vi "Untitled 1.vi"() -> ()   [LabVIEW 2015]
uses:
  <vilib>/measure/NI_MAPro.lvlib
  <vilib>/measure/mamon.llb/Waveform Peak Detection for 1 Chan.vi
  <vilib>/Analysis/NI_AALBase.lvlib
  <vilib>/Analysis/baseanly.llb/Mean (DBL).vi
panel:
  in  "subarray":i32[](array[numeric])
  out "Locations":dbl[](array[numeric]) format="%.2p"
  out "Waveform Chart":i32[](graph)
  out "size(s)":i32
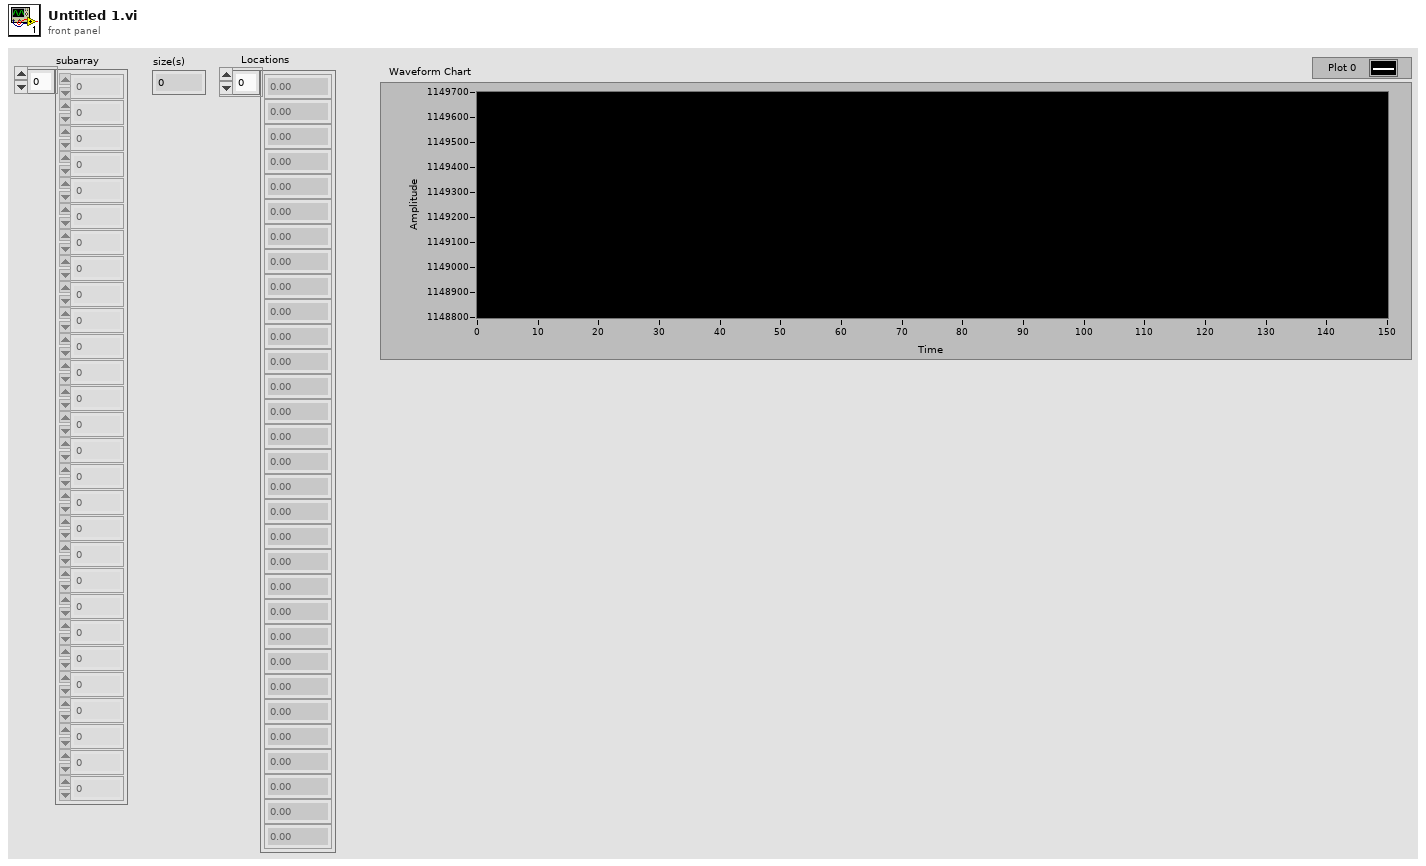
[diagram p1: front panel]
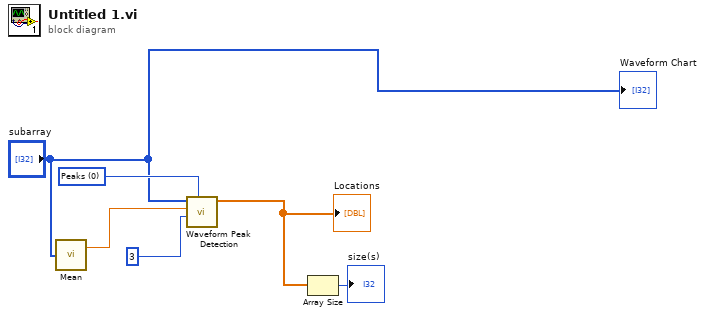
[diagram p0: block diagram]
diagram:
  w4 = u16 0 items=["Peaks", "Valleys"] ("peaks/valleys")
  n1 = call-poly <vilib>:"Mean.vi"("X"="subarray") -> ("mean"=w1:dbl)  [unwired: 1 out]
  n2 = call-poly <vilib>:"Waveform Peak Detection.vi"("peaks/valleys"=w4, "width"=3, "threshold"=w1, "Signal In"="subarray") -> ("Locations"=w5:dbl[])  [unwired: 3 in, 4 out]
  "Locations" <- w5
  n3 = Array Size(array=w5) -> (size(s)=→"size(s)":i32)
  "Waveform Chart" <- "subarray"
